vi "Image Processing-useFIFOtestcomm.vi"() -> ()   [LabVIEW 2016]
uses:
  <vilib>/visionFPGA/Controls/IMAQ FPGA Image Size.ctl
  <vilib>/rvi/Emulation/niFpgaSctlEmulationGetInTimedLoop.vi
  <vilib>/rvi/Emulation/niFpgaProcessEmulError.vi
  <vilib>/rvi/Emulation/niFpgaGetClockAttributes.vi
  <vilib>/rvi/Emulation/niFpgaEmulationReportErrorSimple.vi
  <vilib>/rvi/eio/common/nirviEmuTemplateMethod_errors.vi
  <vilib>/rvi/interface/RandomDataEmulation/niFpgaRandomDataHandleErrors.vi
  <vilib>/rvi/DataTransferAndStorage/Container/Common/niFpgaContainerGetUniqueNameForEmu.vi
  <vilib>/rvi/DataTransferAndStorage/Container/Common/niFpgaContainerSetEmuInfo.vi
  <vilib>/rvi/eio/common/nirviEmuReportErrorAndStop.vi
  <vilib>/rvi/DataTransferAndStorage/Container/Common/niFpgaContainerExecOnDevCompGetState.vi
  <vilib>/rvi/Emulation/niFpgaEmulationIsFPGAContextNoSignature.vi
  <vilib>/rvi/errors/niFpgaSetErrorForExecOnDevCompSimple.vi
  <vilib>/rvi/FIFO/Fifo_Resource/nirvififoEmulationSetSize.vi
  <vilib>/rvi/FIFO/Fifo_Resource/nirviFifoEmulationQueueMgr.vi
  <instcachedir>/0/nirviFifoEmulationQueueMgr_E5CAEC123FF24DC58D834DCA3CDAA9B5.lvgen/nirviFifoEmulationQueueMgr_E5CAEC123FF24DC58D834DCA3CDAA9B5_002.vi
  <vilib>/rvi/FIFO/Fifo_Resource/nirvififoEmulationDetermineInputValidOut.vi
  <vilib>/rvi/FIFO/Fifo_Resource/nirvififoEmulationCreateLock.vi
  <vilib>/rvi/FIFO/Fifo_Resource/nirvififoEmulationObtainLock.vi
  <vilib>/rvi/FIFO/Fifo_Resource/nirvififoEmulationReleaseLock.vi
  <vilib>/rvi/occurrence/nirviWaitOnOccurrenceBase.vi
  <vilib>/rvi/errors/nirviReportUnexpectedCaseInternalError.vi
  <vilib>/rvi/errors/nirviReportUnexpectedCaseInternalError (U32).vi
  <vilib>/Utility/error.llb/Clear Errors.vi
  <vilib>/rvi/Emulation/niFpgaCriticalErrorInLSC.vi
  <vilib>/eio/EIONode/EIONode.xnode
  <vilib>/rvi/DataTransferAndStorage/Container/XNode/niFpgaContainer.xnode
  <vilib>/rvi/interface/RandomDataEmulation/nirviRandomDataFpgaReadWriteTemplate.vi
  <vilib>/rvi/LocalResourceManager/LocalResourceManager.xnode
  <vilib>/rvi/FIFO/Fifo_Resource/niFpgaFifoEmulationRefIn.vi
panel:
  out "CanSendImage":bool=TRUE
  out "Gaussian Out1":u32
  out "In":u32
  out "Mode LED Status":bool=TRUE
  out "Radio LED Status":bool=TRUE
  out "outputExtreme2":bool=TRUE
  out "outputExtreme1":bool=TRUE
  out "outputDOG2":bool=TRUE
  out "outputDOG1":bool=TRUE
  out "outputGaussian2":bool=TRUE
  out "outputGaussian1":bool=TRUE
  out "Ready For Output":bool=TRUE
  out "StartOfImage":bool=TRUE
  in  "Image Size":T1={"Width"=640, "Height"=480}
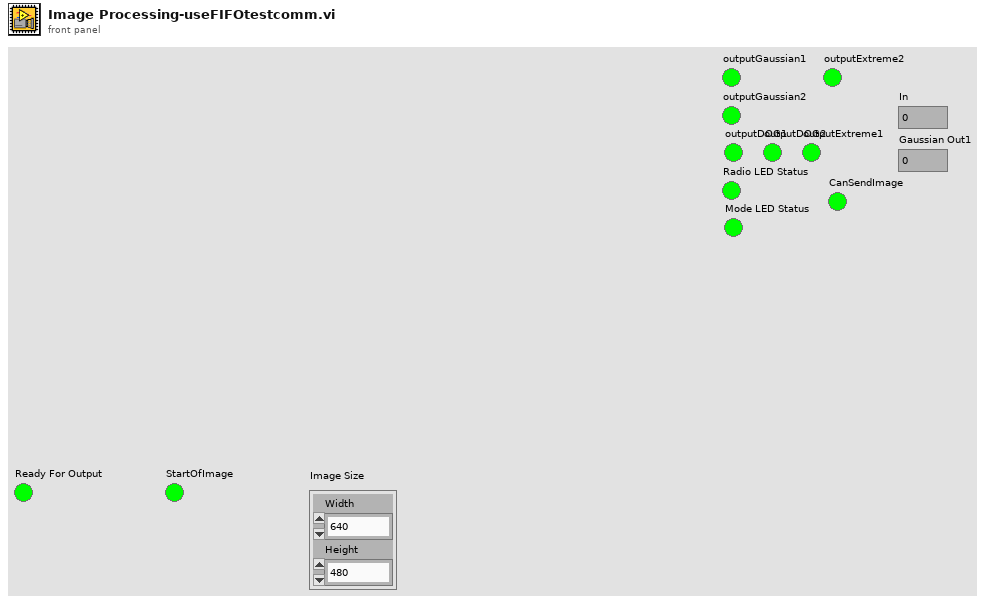
[diagram p1: front panel]
types:
  T1 = typedef "IMAQ FPGA Image Size.ctl" = cluster{"Width":u32, "Height":u32}
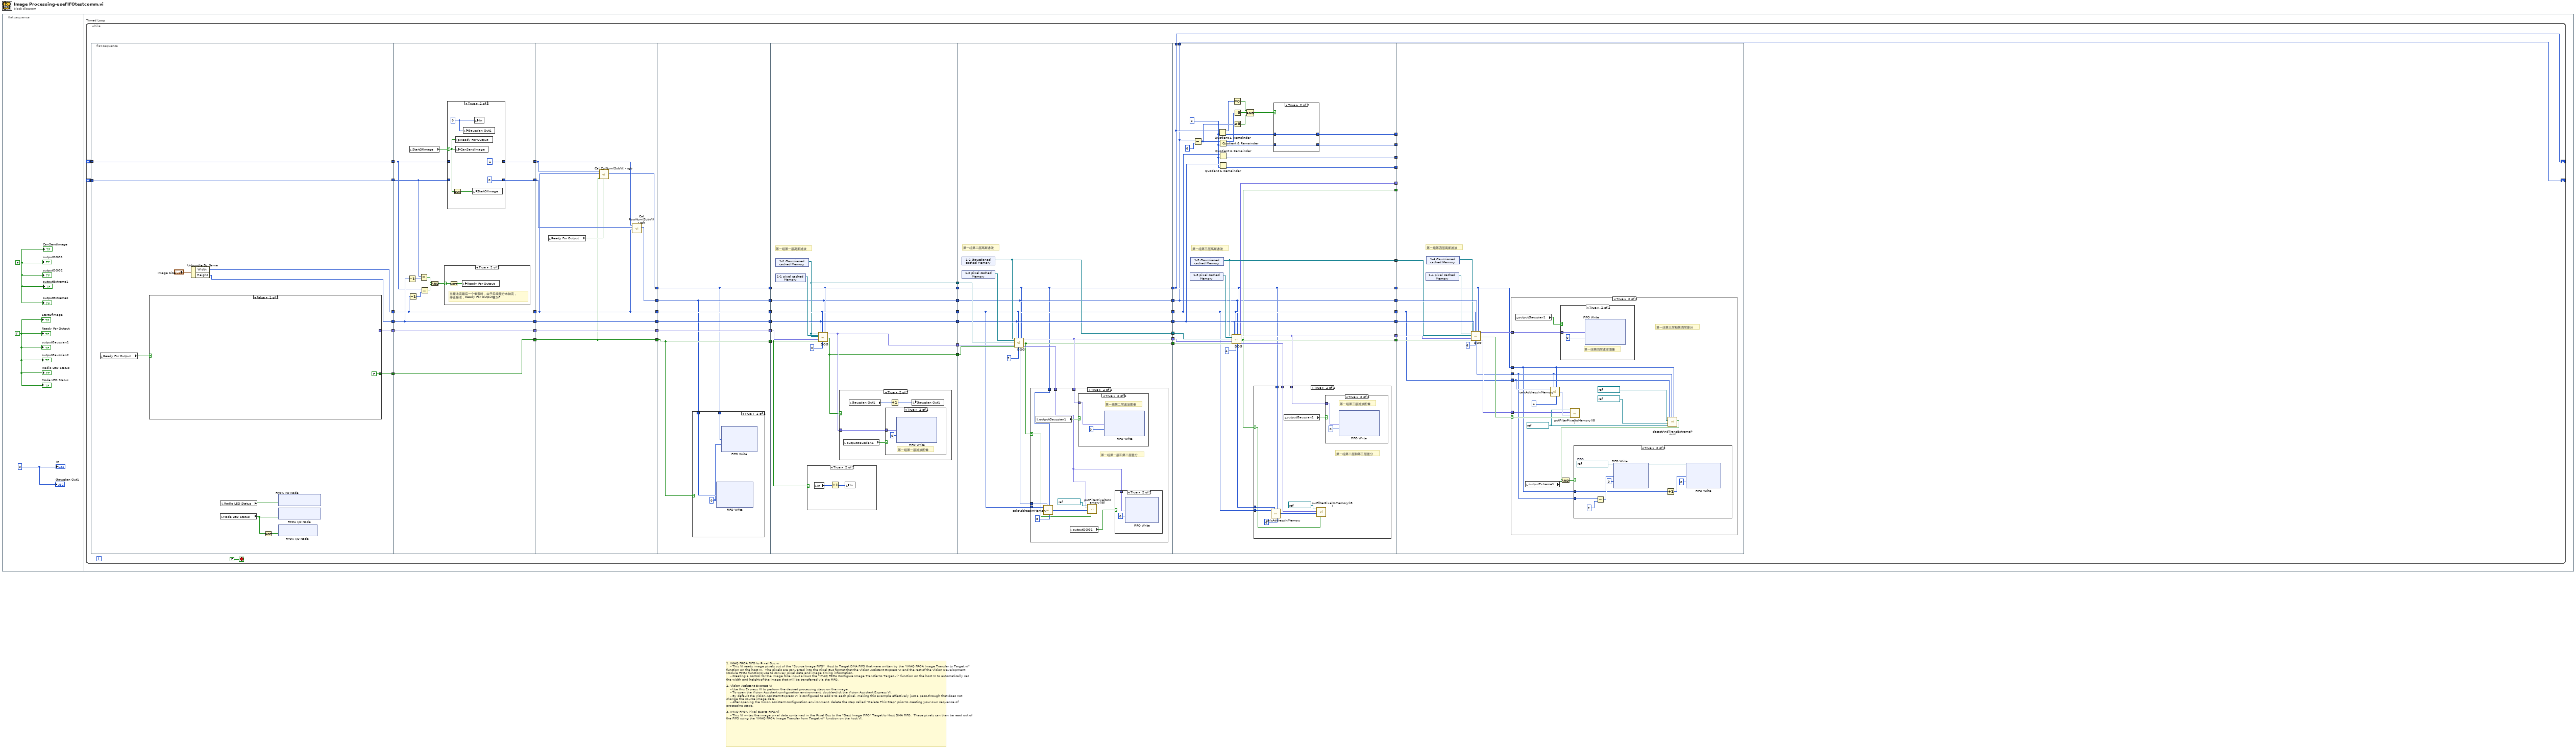
[diagram p0: block diagram]
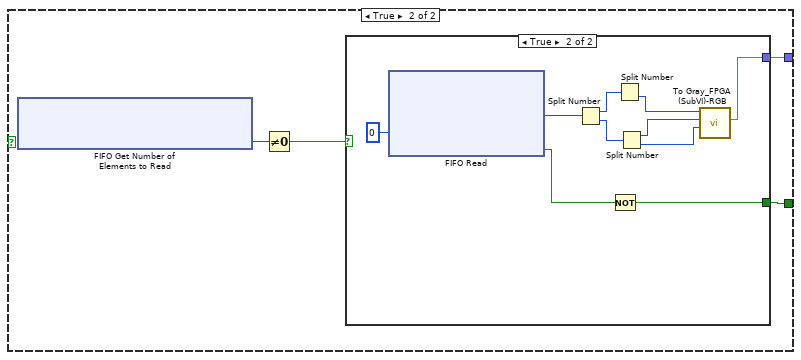
[diagram p2: hidden frame]
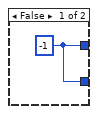
[diagram p13: hidden frame]
diagram:
  # "1. IMAQ FPGA FIFO to Pixel Bus.vi\n    - This VI reads image pixels out of the \"Source Image FIFO\"  Host to Target DMA FIFO that were written by the \"IMAQ FPGA Image Transfer to Target.vi\" function on the host VI.  The pixels are converted into the Pixel Bus format that the Vision Assistant Express VI and the rest of the Vision Development Module FPGA functions use to convey pixel data and image timing information.\n    - Creating a control for the Image Size input allows the \"IMAQ FPGA Configure Image Transfer to Target.vi\" function on the host VI to automatically set the width and height of the image that will be transferred via the FIFO.\n\n2. Vision Assistant Express VI\n    - Use this Express VI to perform the desired processing steps on the image.\n    - To open the Vision Assistant configuration environment, double-click the Vision Assistant Express VI.\n    - By default the Vision Assistant Express VI is configured to add 0 to each pixel, making this example effectively just a pass-through that does not change the source image data.\n    - After opening the Vision Assistant configuration environment, delete the step called \"Delete This Step\" prior to creating your own sequence of processing steps.\n\n3. IMAQ FPGA Pixel Bus to FIFO.vi\n    - This VI writes the image pixel data contained in the Pixel Bus to the \"Dest Image FIFO\" Target to Host DMA FIFO.  These pixels can then be read out of the FIFO using the \"IMAQ FPGA Image Transfer from Target.vi\" function on the host VI."
  n1 = flat-sequence {
    frame #0 {
      w1 = FALSE
      w3 = i16 0
      w2 = TRUE ("Ready For Output")
      "StartOfImage" <- w2
      "Ready For Output" <- w2
      "outputGaussian1" <- w2
      "outputGaussian2" <- w2
      "outputDOG1" <- w1
      "outputDOG2" <- w1
      "outputExtreme1" <- w1
      "outputExtreme2" <- w1
      "Radio LED Status" <- w2
      "Mode LED Status" <- w2
      "In" <- w3
      "Gaussian Out1" <- w3
      "CanSendImage" <- w1
    }
    frame #1 {
      n2 = while "Timed Loop" {
        shift-right: [w4] -> _
        shift-left: _ -> [w9]
        shift-right: [w5] -> _
        shift-left: _ -> [w11]
        stop <- FALSE stop-if-true
        n3 = flat-sequence {
          tunnel: [w61] -> w16
          tunnel: [w60] -> w15
          tunnel: [w67] -> w14
          tunnel: [w66] -> w13
          tunnel: [w65] -> w12
          tunnel: w11 -> [w65]
          tunnel: [w64] -> w10
          tunnel: w9 -> [w64]
          tunnel: [w95] -> w21
          tunnel: [w93] -> w20
          tunnel: [w92] -> w19
          tunnel: [w94] -> w18
          tunnel: w16 -> [w93]
          tunnel: w15 -> [w92]
          tunnel: w14 -> [w95]
          tunnel: w13 -> [w94]
          tunnel: w12 -> [w90]
          tunnel: w10 -> [w88]
          tunnel: [w89] -> w8
          tunnel: [w87] -> w7
          tunnel: [w111] -> w26
          tunnel: [w118] -> w25
          tunnel: [w112] -> w24
          tunnel: [w117] -> w23
          tunnel: [w113] -> w22
          tunnel: w21 -> [w118]
          tunnel: w20 -> [w112]
          tunnel: w19 -> [w117]
          tunnel: w18 -> [w113]
          tunnel: w8 -> [w115]
          tunnel: w7 -> [w116]
          tunnel: [w110] -> w6
          tunnel: [w121] -> w59
          tunnel: [w124] -> w58
          tunnel: [w122] -> w57
          tunnel: [w123] -> w56
          tunnel: [w119] -> w55
          tunnel: [w120] -> w54
          tunnel: w26 -> [w120]
          tunnel: w25 -> [w124]
          tunnel: w24 -> [w123]
          tunnel: w23 -> [w122]
          tunnel: w22 -> [w121]
          tunnel: w6 -> [w119]
          tunnel: w59 -> [w128]
          tunnel: w58 -> [w138]
          tunnel: w57 -> [w134]
          tunnel: w56 -> [w135]
          tunnel: w55 -> [w130]
          tunnel: w54 -> [w129]
          tunnel: [w130] -> w53
          tunnel: [w129] -> w52
          tunnel: [w135] -> w51
          tunnel: [w134] -> w50
          tunnel: [w137] -> w49
          tunnel: [w131] -> w48
          tunnel: [w132] -> w45
          tunnel: w53 -> [w147]
          tunnel: w52 -> [w153]
          tunnel: w51 -> [w149]
          tunnel: w50 -> [w155]
          tunnel: w49 -> [w157]
          tunnel: w48 -> [w156]
          tunnel: [w150] -> w47
          tunnel: [w152] -> w46
          tunnel: w45 -> [w158]
          tunnel: [w147] -> w44
          tunnel: [w153] -> w43
          tunnel: [w149] -> w42
          tunnel: [w155] -> w41
          tunnel: [w154] -> w33
          tunnel: w47 -> [w204]
          tunnel: w46 -> [w203]
          tunnel: w44 -> [w177]
          tunnel: w43 -> [w176]
          tunnel: w42 -> [w178]
          tunnel: w41 -> [w196]
          tunnel: [w182] -> w40
          tunnel: [w180] -> w39
          tunnel: [w177] -> w38
          tunnel: [w176] -> w37
          tunnel: [w178] -> w36
          tunnel: [w196] -> w35
          tunnel: [w201] -> w34
          tunnel: w33 -> [w200]
          tunnel: [w197] -> w32
          tunnel: [w194] -> w31
          tunnel: [w188] -> w30
          tunnel: [w189] -> w29
          tunnel: [w182] -> w28
          tunnel: [w180] -> w27
          tunnel: [w177] -> w5
          tunnel: [w176] -> w4
          tunnel: w40 -> [w233]
          tunnel: w39 -> [w232]
          tunnel: w38 -> [w220]
          tunnel: w37 -> [w231]
          tunnel: w36 -> [w222]
          tunnel: w35 -> [w230]
          tunnel: w34 -> [w227]
          tunnel: w32 -> [_]
          tunnel: w31 -> [_]
          tunnel: w30 -> [_]
          tunnel: w29 -> [_]
          tunnel: w28 -> [_]
          tunnel: w27 -> [_]
          frame #0 {
            n4 = local read "Ready For Output"() -> (w63:bool)
            n5 = case shown="False" w63 {
              tunnel: [_ w73] -> w67
              tunnel: [FALSE w72] -> w66
              frame False {
              }
              frame True {
                n6 = xnode ("FIFO Get Number of Elements to Read")() -> ("Number of Elements to Read"=w75:u32)  [unwired: 1 in, 1 out]
                n7 = Not Equal To 0?(x=w75) -> (x != 0?=w74:bool)
                n8 = case shown="True" w74 {
                  selector: w74 -> [w76 _]
                  tunnel: [_ w79] -> w73
                  tunnel: [w76 w77] -> w72
                  frame False {
                  }
                  frame True {
                    n9 = xnode ("FIFO Read")("Timeout"=0) -> ("Element"=w86:u32, "Timed Out?"=w78:bool)  [unwired: 1 in, 1 out]
                    n10 = Split Number(x=w86) -> (hi(x)=w84:u16, lo(x)=w85:u16)
                    n11 = Not(x=w78) -> (.not. x?=w77:bool)
                    n12 = Split Number(x=w84) -> (lo(x)=w83:u8)  [unwired: 1 out]
                    n13 = Split Number(x=w85) -> (hi(x)=w82:u8, lo(x)=w81:u8)
                    n14 = call "To Gray_FPGA (SubVI)-RGB.vi"("B"=w81, "G"=w82, "R"=w83) -> ("Data Out"=w79:fxp<+,8,8>)  [unwired: 8 in]
                  }
                }
              }
            }
            n15 = Unbundle By Name("Image Size") -> ("Width"=w61:u32, "Height"=w60:u32)
            n16 = local read "Mode LED Status"() -> (w70:bool)
            n17 = local read "Radio LED Status"() -> (w68:bool)
            n18 = Not(x=w70) -> (.not. x?=w69:bool)
            n19 = xnode "FPGA I/O Node"("Radio LED Green"=w68) -> ()  [unwired: 1 in, 1 out]
            n20 = xnode "FPGA I/O Node"("Mode LED Green"=w70) -> ()  [unwired: 1 in, 1 out]
            n21 = xnode "FPGA I/O Node"("Mode LED Red"=w69) -> ()  [unwired: 1 in, 1 out]
          }
          frame #1 {
            n22 = Decrement(x=w92) -> (x-1=w98:u32)
            n23 = Decrement(x=w93) -> (x-1=w97:u32)
            n24 = local read "StartOfImage"() -> (w91:bool)
            n25 = Equal?(x=w88, y=w98) -> (x = y?=w100:bool)
            n26 = Equal?(x=w90, y=w97) -> (x = y?=w99:bool)
            n27 = And(x=w100, y=w99) -> (x .and. y?=w96:bool)
            n28 = case shown="True" w96 {
              selector: w96 -> [_ w109]
              frame False {
              }
              frame True {
                # "当接收完最后一个像素时，由于后续差分未做完，\n停止接收，Ready For Output置为F"
                n29 = Not(x=w109) -> (.not. x?=w108:bool)
                n30 = local write "Ready For Output"(w108) -> ()
              }
            }
            n31 = case shown="True" w91 {
              selector: w91 -> [_ w104]
              tunnel: w90 -> [w102 _]
              tunnel: [w102 i16 -1] -> w89
              tunnel: w88 -> [w101 _]
              tunnel: [w101 u16 0 ("curRow")] -> w87
              frame False {
              }
              frame True {
                w107 = u32 0 ("In")
                n32 = Not(x=w104) -> (.not. x?=w103:bool)
                n33 = local write "Ready For Output"(w104) -> ()
                n34 = local write "CanSendImage"(w104) -> ()
                n35 = local write "Gaussian Out1"(w107) -> ()
                n36 = local write "StartOfImage"(w103) -> ()
                n37 = local write "In"(w107) -> ()
              }
            }
          }
          frame #2 {
            n38 = local read "Ready For Output"() -> (w114:bool)
            n39 = call "Cal ColNum(SubVI) - rgb.vi"("Ready For Input"=w114, "DV"=w113, "Width"=w112, "preCol"=w115) -> ("curCol"=w110:u16)  [unwired: 7 in]
            n40 = call "Cal RowNum(SubVI) - rgb.vi"("Width"=w112, "preRow"=w116, "preCol"=w115) -> ("curRow"=w111:u16)  [unwired: 8 in]
          }
          frame #3 {
            n41 = case shown="True" w121 {
              tunnel: w120 -> [_ w127]
              tunnel: w119 -> [_ w126]
              frame False {
              }
              frame True {
                w125 = 0 ("Timeout")
                n42 = xnode ("FIFO Write")("Element"=w127, "Timeout"=w125) -> ()  [unwired: 1 in, 2 out]
                n43 = xnode ("FIFO Write")("Element"=w126, "Timeout"=w125) -> ()  [unwired: 1 in, 2 out]
              }
            }
          }
          frame #4 {
            # "第一组第一层高斯滤波"
            n44 = xnode "1-1 Gaussianed cached Memory"() -> ("Memory Out"=w132:refnum<k21>)
            n45 = xnode "1-1 pixel cached Memory"() -> ("Memory Out"=w136:refnum<k21>)
            n46 = case shown="True" w128 {
              frame False {
              }
              frame True {
                n47 = local read "In"() -> (w140:u32)
                n48 = Increment(x=w140) -> (x+1=w139:u32)
                n49 = local write "In"(w139) -> ()
              }
            }
            n50 = call "DOG.vi"("Gaussianed cached Memory"=w132, "pixel cached Memory"=w136, "preGaussianed cached Memory"=w132, "Data in"=w138, "DV in"=w128, "Height"=w134, "Width"=w135, "DelayRowCount"=i16 0, "Rows"=w129, "Cols"=w130) -> ("GaussianFilterData out"=w137:fxp<+,12,12>, "DV out"=w131:bool)  [unwired: 6 in, 2 out]
            n51 = case shown="True" w131 {
              tunnel: w137 -> [_ w144]
              frame False {
              }
              frame True {
                n52 = local read "outputGaussian1"() -> (w143:bool)
                n53 = local read "Gaussian Out1"() -> (w141:u32)
                n54 = case shown="True" w143 {
                  tunnel: w144 -> [_ w145]
                  frame False {
                  }
                  frame True {
                    # "第一组第一层滤波图像"
                    n55 = xnode ("FIFO Write")("Element"=w145, "Timeout"=0) -> ()  [unwired: 1 in, 2 out]
                  }
                }
                n56 = Increment(x=w141) -> (x+1=w142:u32)
                n57 = local write "Gaussian Out1"(w142) -> ()
              }
            }
          }
          frame #5 {
            # "第一组第二层高斯滤波"
            n58 = xnode "1-2 Gaussianed cached Memory"() -> ("Memory Out"=w154:refnum<k21>)
            n59 = xnode "1-2 pixel cached Memory"() -> ("Memory Out"=w159:refnum<k21>)
            n60 = call "DOG.vi"("Gaussianed cached Memory"=w154, "pixel cached Memory"=w159, "preGaussianed cached Memory"=w158, "Data in"=w157, "DV in"=w156, "Height"=w155, "Width"=w149, "DelayRowCount"=i16 2, "Rows"=w153, "Cols"=w147) -> ("out Row"=w148:u16, "GaussianFilterData out"=w152:fxp<+,12,12>, "DV out"=w150:bool, "DOG Out"=w151:fxp<+/-,13,13>)  [unwired: 6 in]
            n61 = case shown="True" w150 {
              selector: w150 -> [_ w164]
              tunnel: w152 -> [_ w171]
              tunnel: w151 -> [_ w162]
              tunnel: w149 -> [_ w170]
              tunnel: w148 -> [_ w169]
              tunnel: w147 -> [_ w168]
              frame False {
              }
              frame True {
                # "第一组第一层和第二层差分"
                n62 = local read "outputGaussian1"() -> (w163:bool)
                n63 = call "calcAddressInMemory.vi"("Width"=w170, "Rows"=w169, "Cols"=w168, "divider"=u8 8) -> ("addressInMemory"=w166:u16)  [unwired: 5 in]
                n64 = local read "outputDOG1"() -> (w161:bool)
                n65 = case shown="True" w163 {
                  tunnel: w171 -> [_ w174]
                  frame False {
                  }
                  frame True {
                    # "第一组第二层滤波图像"
                    n66 = xnode ("FIFO Write")("Element"=w174, "Timeout"=0) -> ()  [unwired: 1 in, 2 out]
                  }
                }
                n67 = call "putFilterPixeltoMemory(I8).vi"("DV in"=w164, "addressInMemory"=w166, "Data In"=w162, "Memory in"=refnum<k21> "DOG1-1") -> ()  [unwired: 8 in]
                n68 = case shown="True" w161 {
                  tunnel: w162 -> [_ w173]
                  frame False {
                  }
                  frame True {
                    n69 = xnode ("FIFO Write")("Element"=w173, "Timeout"=0) -> ()  [unwired: 1 in, 2 out]
                  }
                }
              }
            }
          }
          frame #6 {
            w195 = u32 2 ("y")
            # "第一组第三层高斯滤波"
            n70 = xnode "1-3 pixel cached Memory"() -> ("Memory Out"=w202:refnum<k21>)
            n71 = xnode "1-3 Gaussianed cached Memory"() -> ("Memory Out"=w201:refnum<k21>)
            n72 = Subtract(x=w176, y=i16 6) -> (x-y=w185:u16)
            n73 = Quotient & Remainder(x=w177, y=w195) -> (x-y*floor(x/y)=w184:u32, floor(x/y)=w186:u32)
            n74 = Quotient & Remainder(x=w185, y=w195) -> (x-y*floor(x/y)=w183:u32, floor(x/y)=w187:u32)
            n75 = Quotient & Remainder(x=w178, y=w195) -> (floor(x/y)=w197:u32)  [unwired: 1 out]
            n76 = Quotient & Remainder(x=w196, y=w195) -> (floor(x/y)=w194:u32)  [unwired: 1 out]
            n77 = call "DOG.vi"("Gaussianed cached Memory"=w201, "pixel cached Memory"=w202, "preGaussianed cached Memory"=w200, "Data in"=w203, "DV in"=w204, "Height"=w196, "Width"=w178, "DelayRowCount"=i16 4, "Rows"=w176, "Cols"=w177) -> ("out Row"=w179:u16, "GaussianFilterData out"=w182:fxp<+,12,12>, "DV out"=w180:bool, "DOG Out"=w181:fxp<+/-,13,13>)  [unwired: 6 in]
            n78 = Equal To 0?(x=w184) -> (x = 0?=w193:bool)
            n79 = Equal To 0?(x=w183) -> (x = 0?=w192:bool)
            n80 = Greater Or Equal To 0?(x=w185) -> (x >= 0?=w191:bool)
            n81 = Compound Arithmetic op=AND(w193, w192, w191) -> (w190:bool)
            n82 = case shown="True" w180 {
              selector: w180 -> [_ w209]
              tunnel: w182 -> [_ w217]
              tunnel: w181 -> [_ w210]
              tunnel: w179 -> [_ w213]
              tunnel: w178 -> [_ w212]
              tunnel: w177 -> [_ w211]
              frame False {
              }
              frame True {
                # "第一组第二层和第三层差分"
                n83 = call "calcAddressInMemory.vi"("Width"=w212, "Rows"=w213, "Cols"=w211, "divider"=u8 6) -> ("addressInMemory"=w215:u16)  [unwired: 5 in]
                n84 = local read "outputGaussian1"() -> (w208:bool)
                n85 = call "putFilterPixeltoMemory(I8).vi"("DV in"=w209, "addressInMemory"=w215, "Data In"=w210, "Memory in"=refnum<k21> "DOG1-2") -> ()  [unwired: 8 in]
                n86 = case shown="True" w208 {
                  tunnel: w217 -> [_ w218]
                  frame False {
                  }
                  frame True {
                    # "第一组第三层滤波图像"
                    n87 = xnode ("FIFO Write")("Element"=w218, "Timeout"=0) -> ()  [unwired: 1 in, 2 out]
                  }
                }
              }
            }
            n88 = case shown="True" w190 {
              tunnel: [w205 w207] -> w189
              tunnel: w186 -> [_ w207]
              tunnel: [w205 w206] -> w188
              tunnel: w187 -> [_ w206]
              frame False {
                w205 = i16 -1 ("t")
              }
              frame True {
              }
            }
          }
          frame #7 {
            # "第一组第四层高斯滤波"
            n89 = xnode "1-4 pixel cached Memory"() -> ("Memory Out"=w228:refnum<k21>)
            n90 = xnode "1-4 Gaussianed cached Memory"() -> ("Memory Out"=w229:refnum<k21>)
            n91 = call "DOG.vi"("Gaussianed cached Memory"=w229, "pixel cached Memory"=w228, "preGaussianed cached Memory"=w227, "Data in"=w233, "DV in"=w232, "Height"=w230, "Width"=w222, "DelayRowCount"=i16 6, "Rows"=w231, "Cols"=w220) -> ("out Row"=w221:u16, "GaussianFilterData out"=w225:fxp<+,12,12>, "DV out"=w224:bool, "DOG Out"=w223:fxp<+/-,13,13>)  [unwired: 6 in]
            n92 = case shown="True" w224 {
              selector: w224 -> [_ w244]
              tunnel: w225 -> [_ w248]
              tunnel: w223 -> [_ w245]
              tunnel: w222 -> [_ w243]
              tunnel: w221 -> [_ w237]
              tunnel: w220 -> [_ w238]
              frame False {
              }
              frame True {
                w240 = refnum<k21> "DOG1-3" ("Memory in")
                # "第一组第三层和第四层差分"
                n93 = local read "outputGaussian1"() -> (w239:bool)
                n94 = local read "outputExtreme1"() -> (w235:bool)
                n95 = call "calcAddressInMemory.vi"("Width"=w243, "Rows"=w237, "Cols"=w238, "divider"=u8 4) -> ("addressInMemory"=w246:u16)  [unwired: 5 in]
                n96 = case shown="True" w239 {
                  tunnel: w248 -> [_ w259]
                  frame False {
                  }
                  frame True {
                    # "第一组第四层滤波图像"
                    n97 = xnode ("FIFO Write")("Element"=w259, "Timeout"=0) -> ()  [unwired: 1 in, 2 out]
                  }
                }
                n98 = call "putFilterPixeltoMemory(I8).vi"("DV in"=w244, "addressInMemory"=w246, "Data In"=w245, "Memory in"=w240) -> ()  [unwired: 8 in]
                n99 = call "detectAndTransExtremePoint.vi"("Col"=w238, "Row"=w237, "Level3 Memory"=w240, "Level2 Memory"=refnum<k21> "DOG1-2" ("Memory In"), "Level1 Memory"=refnum<k21> "DOG1-1" ("Memory In"), "Width"=w243) -> ("isExtreme?"=w234:bool)  [unwired: 5 in]
                n100 = And(x=w234, y=w235) -> (x .and. y?=w236:bool)
                n101 = case shown="True" w236 {
                  tunnel: w237 -> [_ w256]
                  tunnel: w238 -> [_ w250]
                  frame False {
                  }
                  frame True {
                    w249 = refnum<k21> "extreme FIFO"  # FIFO
                    n102 = Subtract(x=w256, y=u16 2) -> (x-y=w254:u16)
                    n103 = xnode ("FIFO Write")("Element"=w254, "Timeout"=0, "FIFO In"=w249) -> ("FIFO Out"=w252:refnum<k21>)  [unwired: 1 out]
                    n104 = Increment(x=w250) -> (x+1=w251:u16)
                    n105 = xnode ("FIFO Write")("Element"=w251, "Timeout"=0, "FIFO In"=w252) -> ()  [unwired: 2 out]
                  }
                }
              }
            }
          }
        }
      }
    }
  }
